vi "Build Measurement Query.vi"(8 "error in":errorcluster, 11 "3300 in":refnum<class "3300.lvclass">) -> (0 "error out":errorcluster, 2 "Measurement Query":string, 3 "3300 out":refnum<class "3300.lvclass">)   [LabVIEW 2019, in "3300.lvlib" / "3300.lvclass"]
doc: "Construct Measurement query based on available channels\nQuery the following values in order:\n1. Measure Voltage\n2. Measure Current\n3. Output Enabled\n4. Status Register"
uses:
  Library/3300.lvclass
  C:/Users/Public/Documents/Development/builds/Instruments/Electronic Load.lvlibp/Library/Electronic Load.lvclass
  builds/Instruments/Electronic Load.lvlibp/Accessors/Read Available Channels.vi
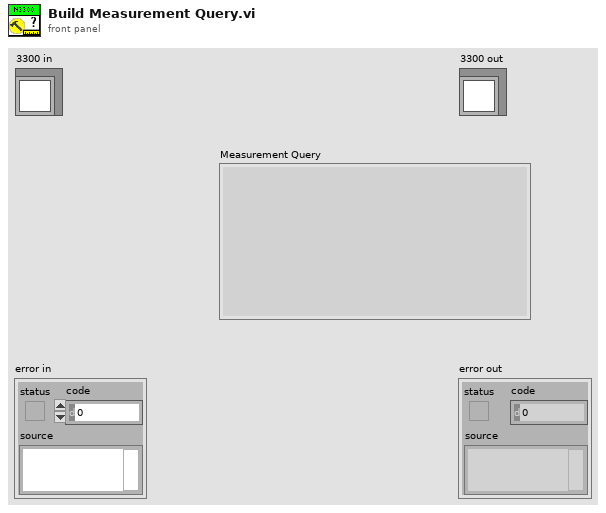
[diagram p1: front panel]
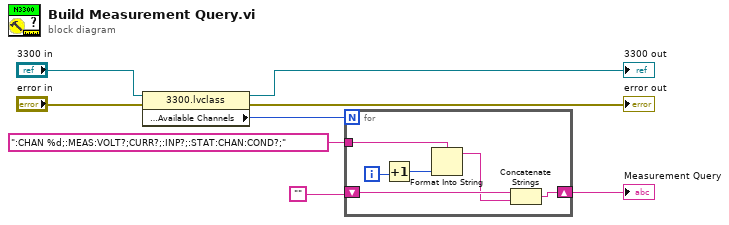
[diagram p0: block diagram]
diagram:
  n1 = property class="3300.lvclass"(reference="3300 in", error in="error in") -> (reference out=→"3300 out":refnum<class "3300.lvclass">, error out=→"error out":errorcluster, "Accessors:Configuration:Available Channels"=w1:i32)
  n2 = for {
    N: w1 -> [_]
    tunnel: ":CHAN %d;:MEAS:VOLT?;CURR?;:INP?;:STAT:CHAN:COND?;" -> [w14]
    shift-right: [w9] -> w6
    shift-left: "" -> [w11]
    i -> [w13]
    n3 = Increment(x=w13) -> (x+1=w12:i32)
    n4 = Format Into String(format string=w14, w12) -> (resulting string=w10:string)  [unwired: 2 in, 1 out]
    n5 = Concatenate Strings(w11, w10) -> (w9:string)
  }
  "Measurement Query" <- w6
